vi "Signal State Controller.vi"(6 "stop":bool, 7 "reset":bool, 8 "error IO":errorcluster, 10 "current time":timestamp, 11 "signal configuration":refnum<class "SV Signal.lvclass">) -> (0 "error out":errorcluster, 1 "waveform dt":dbl, 2 "waveform t0":timestamp, 3 "signal configuration":refnum<class "SV Signal.lvclass">)   [LabVIEW 2017, in "SV Signal.lvclass"]
uses:
  <vilib>/addons/_NISVFA/_Generation/Signal Generation/SV Signal/SV Signal.lvclass
  <vilib>/addons/_NISVFA/_Generation/Signal Generation/SV Signal/SV Signal.lvclass/SV Signal.ctl
  <vilib>/addons/_NISVFA/_Generation/Signal Generation/SV Signal/sv_Signal State Attribute.ctl
  <vilib>/addons/_NISVFA/_Generation/Signal Generation/SV Signal/sv_Generation State.ctl
  <vilib>/addons/_NISVFA/_Generation/subVIs/sv_Optimum Location.ctl
  <vilib>/addons/_NISVFA/_Generation/SoundVib_Generation.lvlib
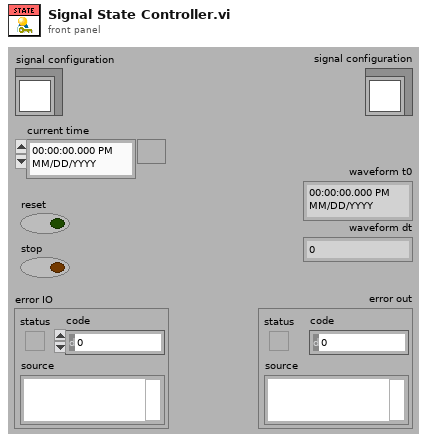
[diagram p1: front panel]
types:
  T1 = typedef "SV Signal.lvclass/sv_Signal State Attribute.ctl" = string
  T2 = typedef "SV Signal.lvclass/sv_Generation State.ctl" = enum16{"Idle", "Ramp Up", "Pre-Measurement Settling", "Measurement", "Post-Measurement Settling", "Discrete Sweep Transition", "Ramp Down", "Update"}
  T3 = typedef "SoundVib_Generation.lvlib/sv_Optimum Location.ctl" = enum16{"Zero Crossing, First Available", "Zero Crossing, Positive Slope", "Zero Crossing, Negative Slope", "Peak or Valley", "Peak", "Valley"}
  T4 = typedef "SV Signal.lvclass/sv_System Timing Model.ctl" = i64
  T5 = cluster{"system timing model":T4, "state":cluster{"RESET":bool, "generator timestamp":timestamp, "elapsed seconds":dbl, "elapsed samples":u64, "generation state":T2, "time offset at state":dbl, "samples generated at state":u64, "signal state":variant}, "duration of state":dbl, "samples remaining at state":i32}
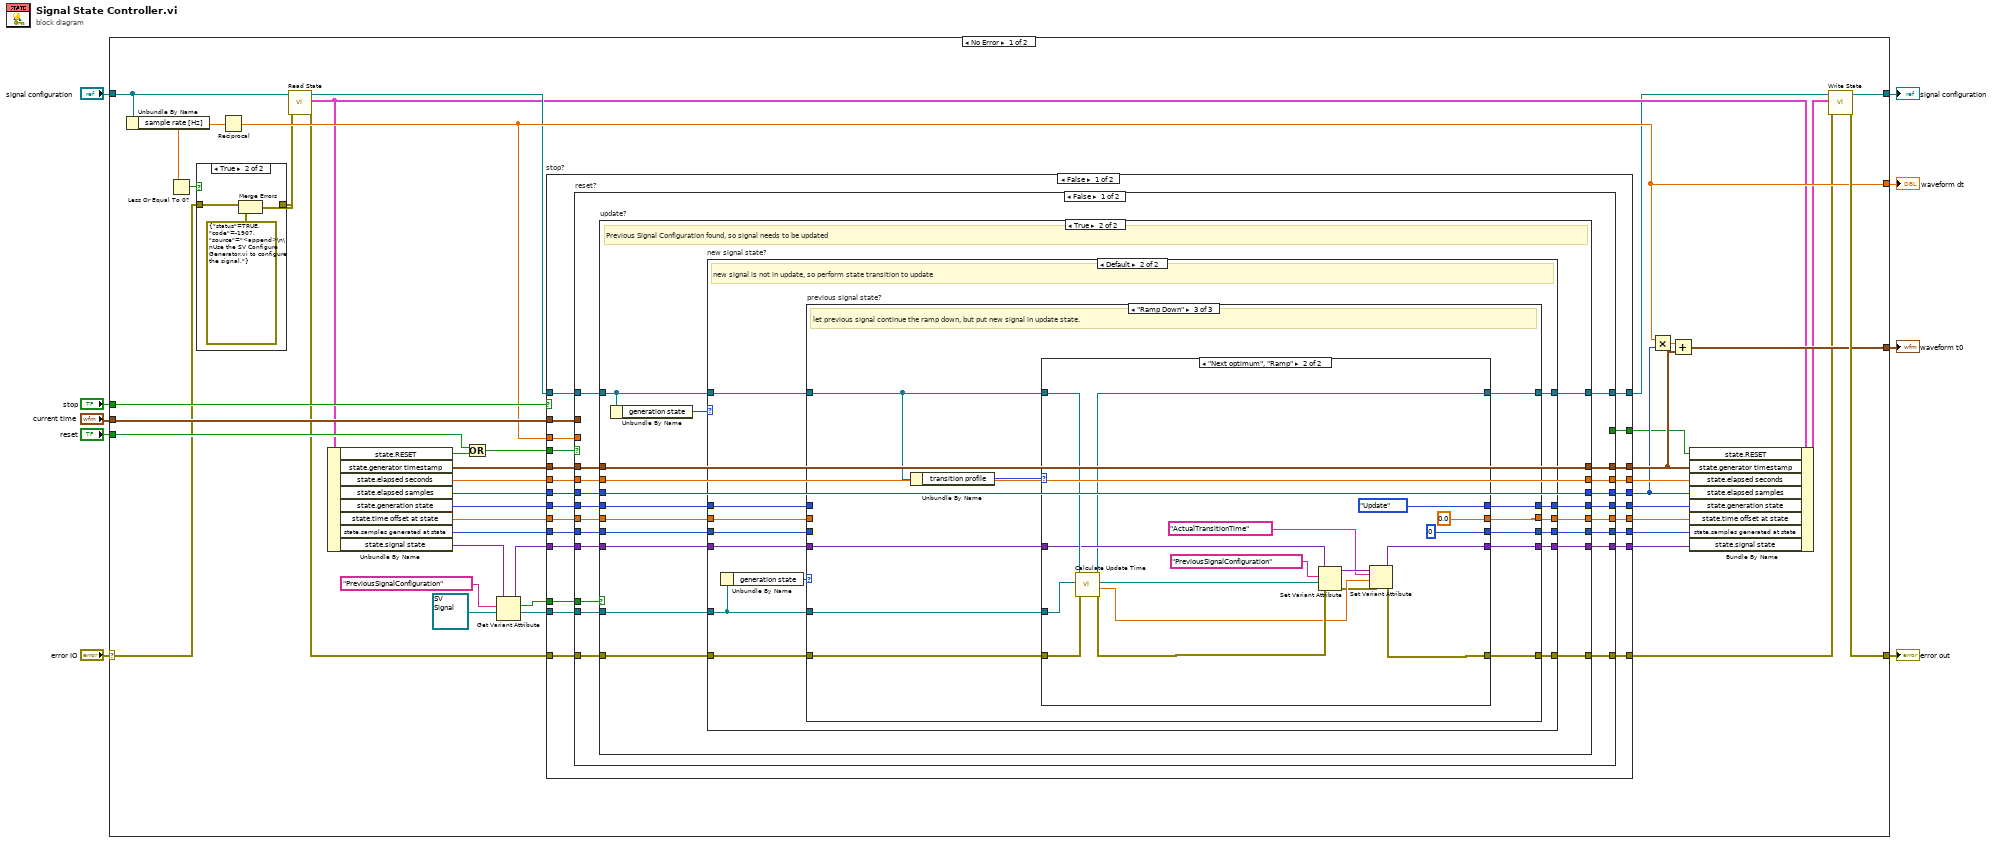
[diagram p0: block diagram]
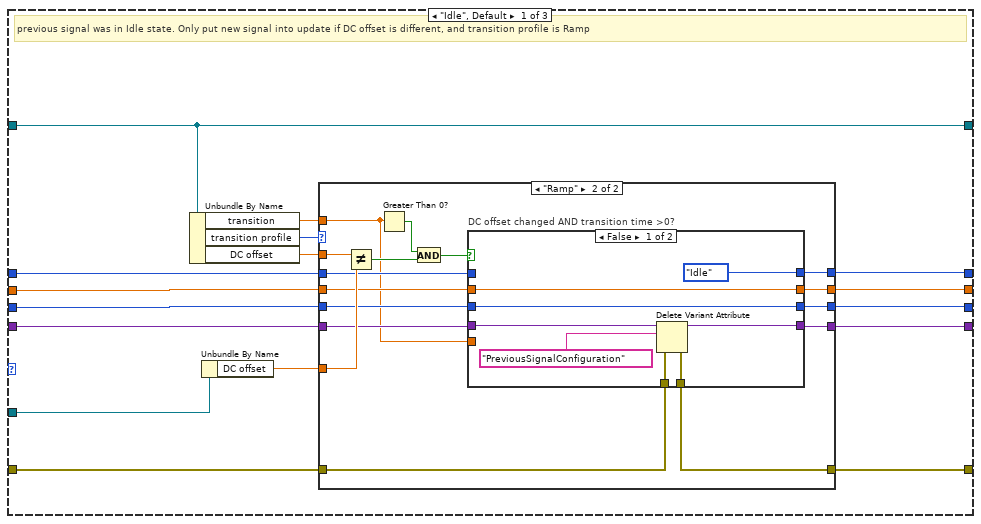
[diagram p5: hidden frame]
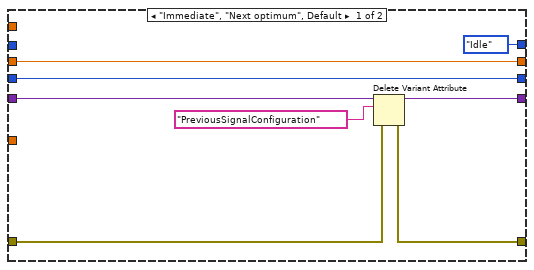
[diagram p6: hidden frame]
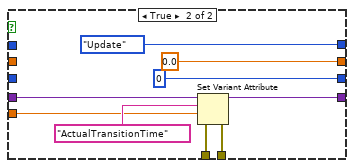
[diagram p7: hidden frame]
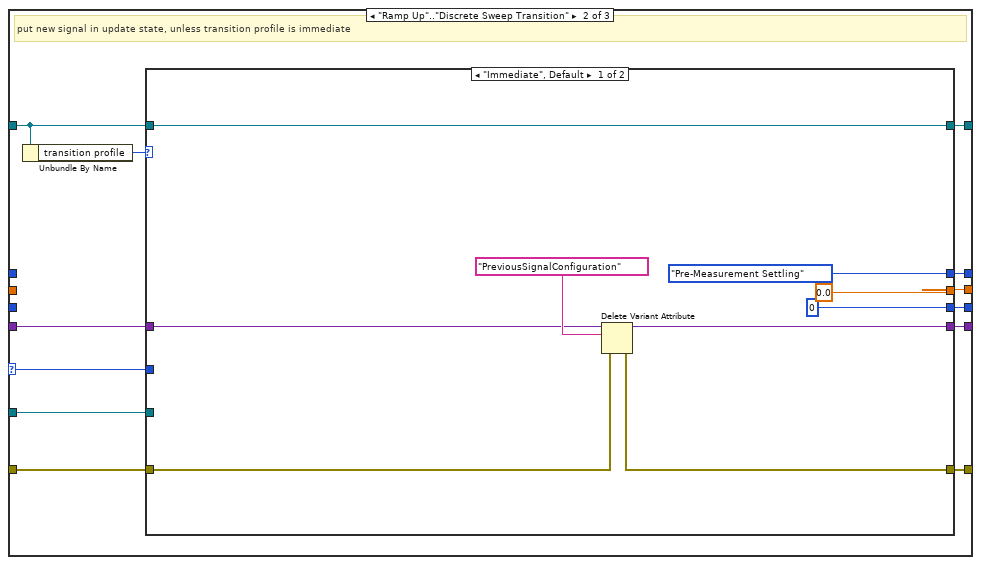
[diagram p8: hidden frame]
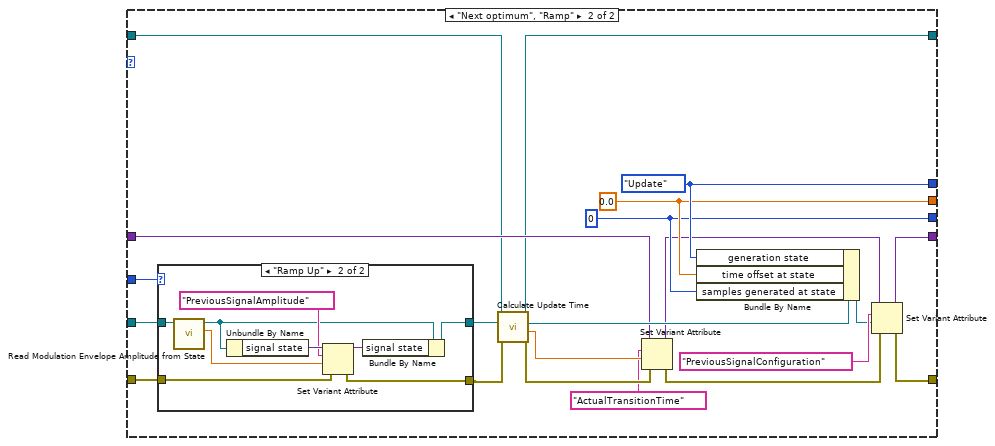
[diagram p9: hidden frame]
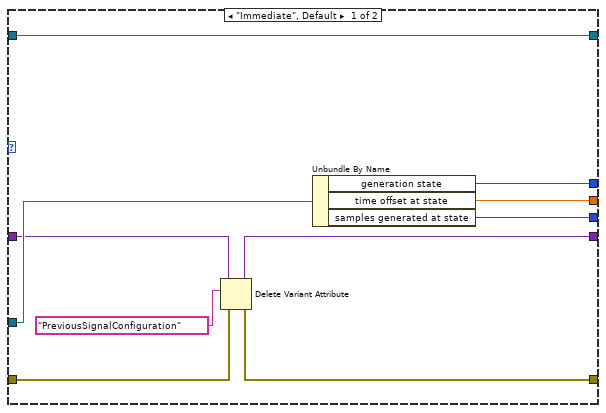
[diagram p11: hidden frame]
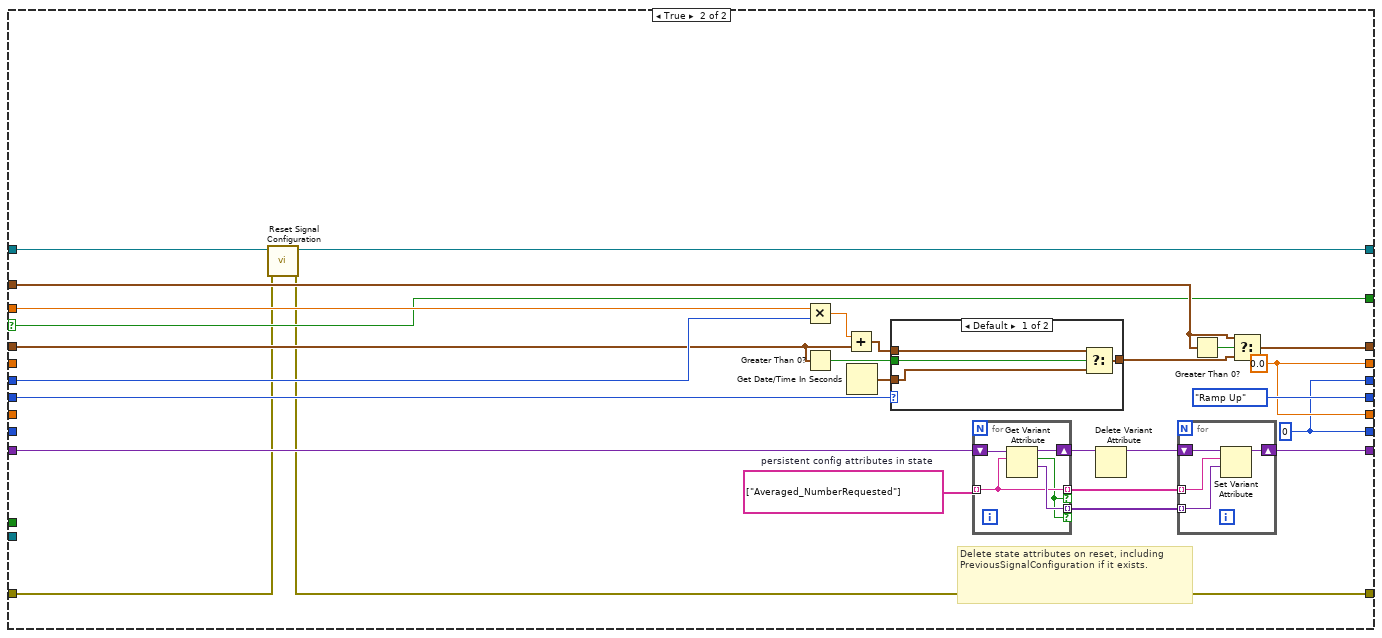
[diagram p12: hidden frame]
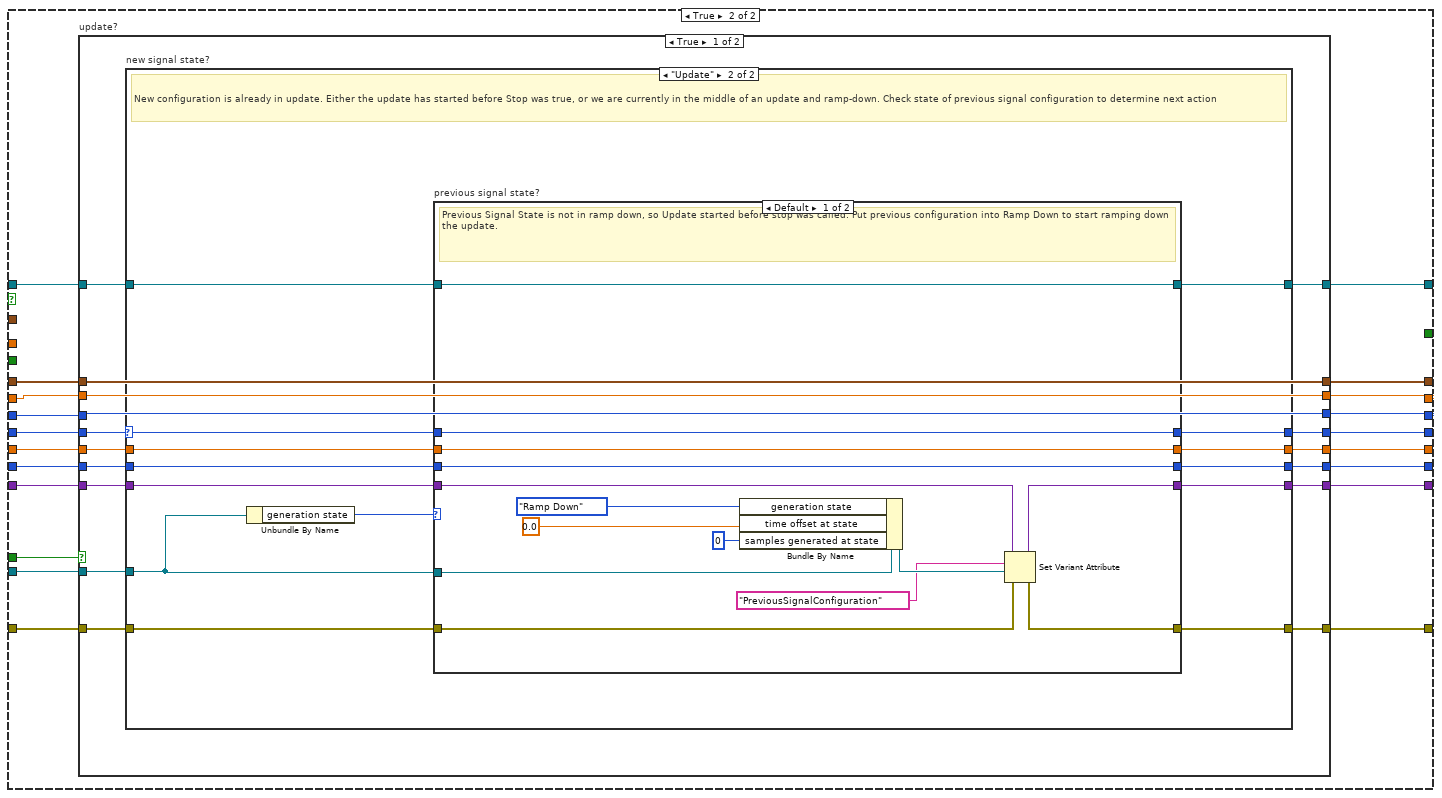
[diagram p14: hidden frame]
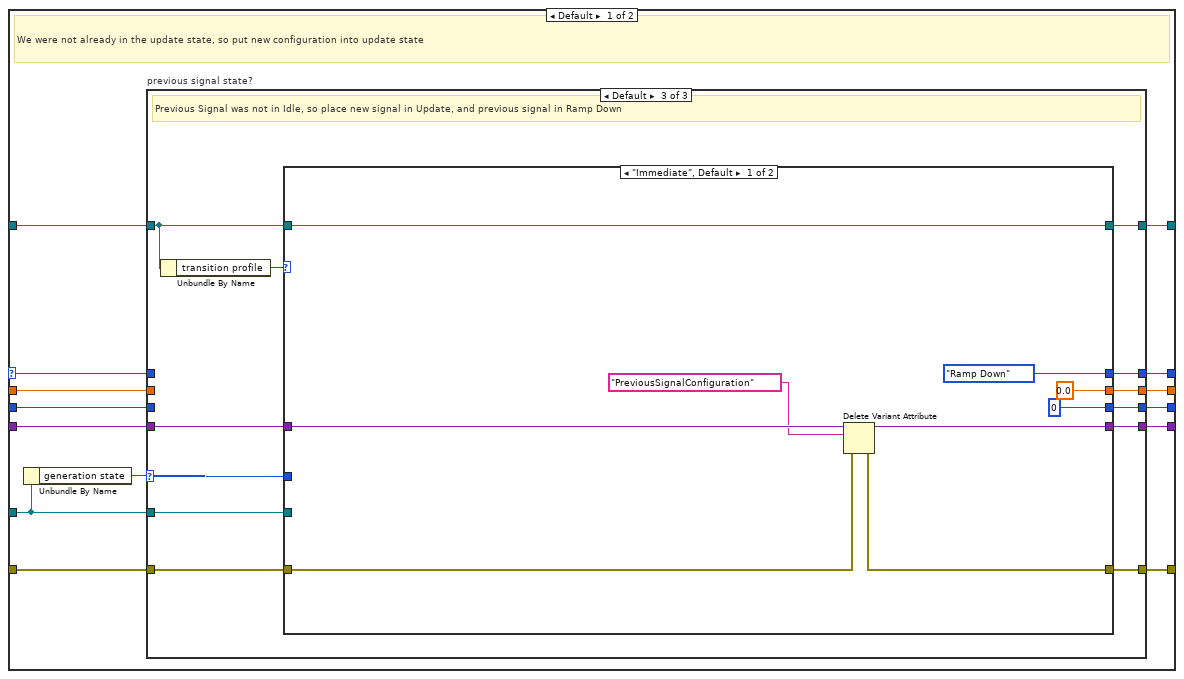
[diagram p15: hidden frame]
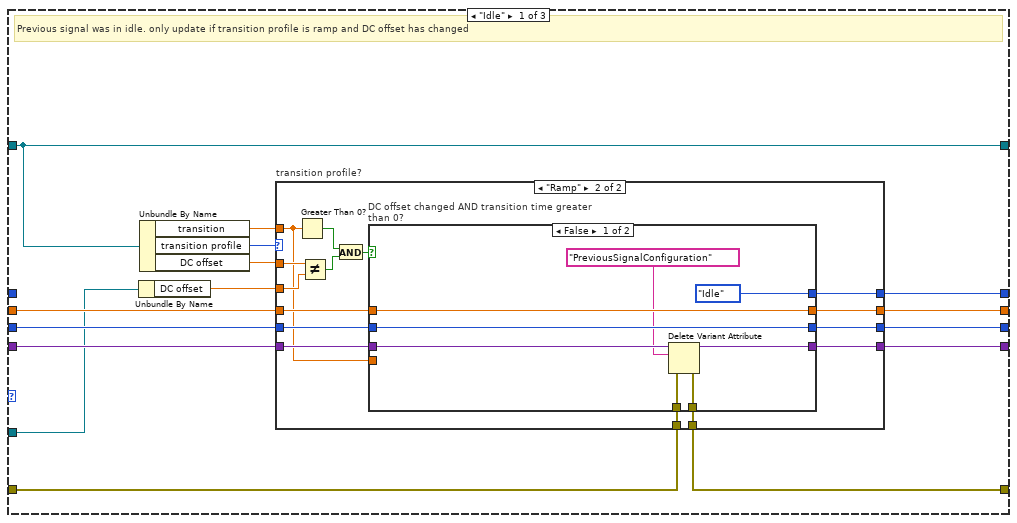
[diagram p16: hidden frame]
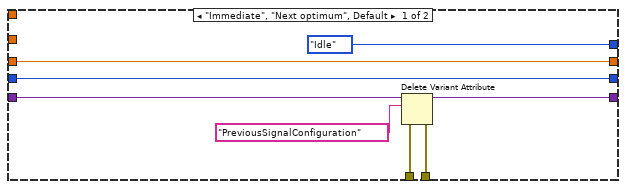
[diagram p17: hidden frame]
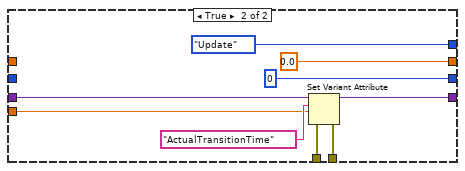
[diagram p18: hidden frame]
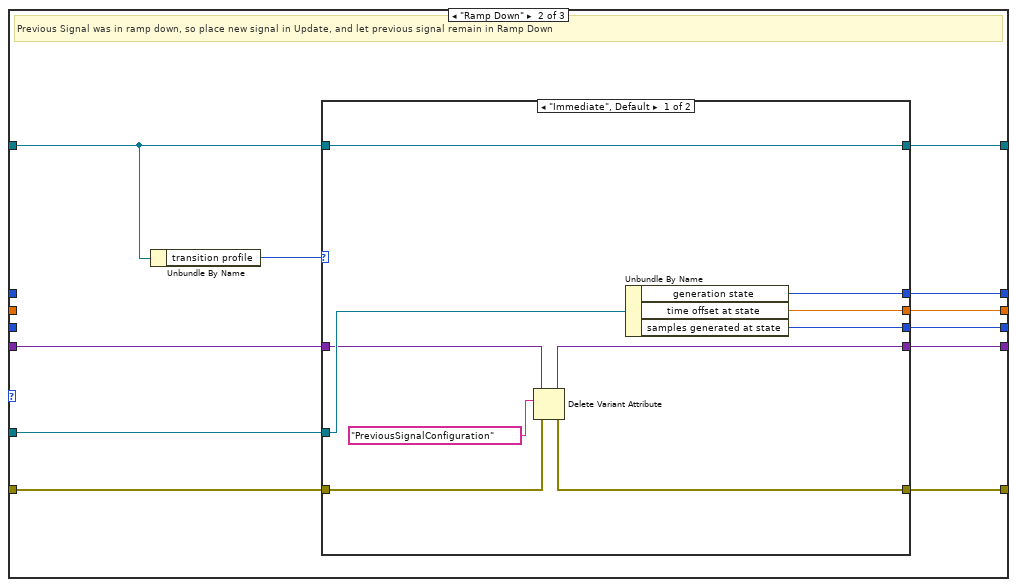
[diagram p19: hidden frame]
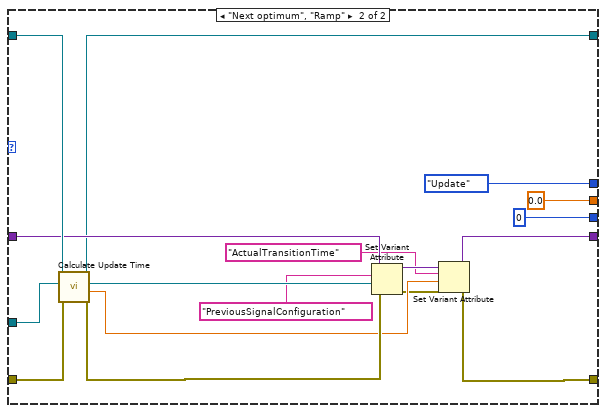
[diagram p20: hidden frame]
diagram:
  n1 = case shown="No Error" "error IO" {
    selector: "error IO" -> [w11 w618]
    tunnel: [w30 _] -> w9
    tunnel: "signal configuration" -> [w13 w619]
    tunnel: [w18 w619] -> w7
    tunnel: [w39 w618] -> w6
    tunnel: "stop" -> [w38 _]
    tunnel: "reset" -> [w36 _]
    tunnel: "current time" -> [w31 _]
    tunnel: [w29 nan] -> w1
    frame No Error {
      n2 = Unbundle By Name(w13) -> ("sample rate [Hz]"=w15:dbl)
      n3 = Less Or Equal To 0?(x=w15) -> (x <= 0?=w14:bool)
      n4 = case shown="True" w14 {
        tunnel: w11 -> [w51 w54]
        tunnel: [w51 w52] -> w10
        frame False {
        }
        frame True {
          n5 = Merge Errors(w54, errorcluster {"status"=TRUE, "code"=-1907, "source"="<append>\n\nUse the SV Configure Generator.vi to configure the signal."} ("error in (no error)")) -> (w52:errorcluster)
        }
      }
      n6 = Reciprocal(x=w15) -> (1/x=w29:dbl)
      n7 = call <vilib>:"Read State.vi"("error in (no error)"=w10, "signal configuration"=w13) -> ("error out"=w12:errorcluster, "generator state"=w20:T5, "signal configuration"=w28:refnum<class "SV Signal.lvclass">)  [unwired: 7 in]
      n8 = Unbundle By Name(w20) -> ("state.RESET"=w37:bool, "state.generator timestamp"=w44:timestamp, "state.elapsed seconds"=w45:dbl, "state.elapsed samples"=w46:u64, "state.generation state"=w47:T2, "state.time offset at state"=w43:dbl, "state.samples generated at state"=w42:u64, "state.signal state"=w25:variant)
      n9 = Or(x=w36, y=w37) -> (x .or. y?=w35:bool)
      n10 = Get Variant Attribute(Variant=w25, name=T1 "PreviousSignalConfiguration", default value (empty Variant)=refnum<class "SV Signal.lvclass"> refnum ("signal configuration")) -> (duplicate Variant=w24:variant, found=w23:bool, value=w22:refnum<class "SV Signal.lvclass">)  [unwired: 1 in, 1 out]
      n11 = case "stop?" shown="False" w38 {
        tunnel: [w78 w340] -> w50
        tunnel: [w77 w342] -> w49
        tunnel: [w76 w353] -> w48
        tunnel: [w75 w338] -> w32
        tunnel: w35 -> [w74 _]
        tunnel: w47 -> [w73 w350]
        tunnel: w46 -> [w72 w337]
        tunnel: w45 -> [w71 w339]
        tunnel: w44 -> [w70 w341]
        tunnel: w43 -> [w69 w349]
        tunnel: w42 -> [w68 w348]
        tunnel: [w67 w352] -> w41
        tunnel: [w66 w351] -> w40
        tunnel: w24 -> [w65 w347]
        tunnel: [w64 w346] -> w34
        tunnel: w31 -> [w63 _]
        tunnel: w29 -> [w62 _]
        tunnel: w28 -> [w57 w345]
        tunnel: w23 -> [w61 w336]
        tunnel: w22 -> [w60 w335]
        tunnel: w12 -> [w59 w343]
        tunnel: [w58 w344] -> w21
        tunnel: [w56 _] -> w17
        tunnel: [w55 w334] -> w16
        frame False {
          n12 = case "reset?" shown="False" w74 {
            selector: w74 -> [_ w297]
            tunnel: w70 -> [w95 w301]
            tunnel: [w96 w315] -> w77
            tunnel: [w94 w318] -> w78
            tunnel: [w92 w317] -> w75
            tunnel: w71 -> [w93 _]
            tunnel: w72 -> [w91 w304]
            tunnel: w73 -> [w89 w302]
            tunnel: [w90 sv_Generation_State."Ramp Up" ("generation state")] -> w76
            tunnel: w69 -> [w87 _]
            tunnel: w68 -> [w85 _]
            tunnel: [w88 w318] -> w67
            tunnel: [w86 w317] -> w66
            tunnel: w65 -> [w83 w309]
            tunnel: [w84 w308] -> w64
            tunnel: w63 -> [_ w314]
            tunnel: w62 -> [_ w305]
            tunnel: w61 -> [w97 _]
            tunnel: w60 -> [w98 _]
            tunnel: w59 -> [w82 w294]
            tunnel: [w81 w293] -> w58
            tunnel: w57 -> [w80 w296]
            tunnel: [_ w297] -> w56
            tunnel: [w79 w295] -> w55
            frame False {
              n13 = case "update?" shown="True" w97 {
                tunnel: w98 -> [_ w120]
                tunnel: [w107 w124] -> w96
                tunnel: w95 -> [w107 w124]
                tunnel: [w106 w123] -> w94
                tunnel: w93 -> [w106 w123]
                tunnel: [w105 w122] -> w92
                tunnel: w91 -> [w105 w122]
                tunnel: [w104 w114] -> w90
                tunnel: w89 -> [w104 w118]
                tunnel: [w103 w113] -> w88
                tunnel: w87 -> [w103 w117]
                tunnel: [w102 w112] -> w86
                tunnel: w85 -> [w102 w116]
                tunnel: [w101 w111] -> w84
                tunnel: w83 -> [w101 w115]
                tunnel: w82 -> [w100 w121]
                tunnel: [w100 w119] -> w81
                tunnel: w80 -> [w99 w110]
                tunnel: [w99 w108] -> w79
                frame False {
                  # "No previous signal configuration found, don't update signal state"
                }
                frame True {
                  # "Previous Signal Configuration found, so signal needs to be updated"
                  n14 = Unbundle By Name(w110) -> ("generation state"=w109:T2)
                  n15 = case "new signal state?" shown="Default" w109 {
                    tunnel: w121 -> [w130 w143]
                    tunnel: w120 -> [_ w142]
                    tunnel: [w130 w141] -> w119
                    tunnel: [w126 w140] -> w114
                    tunnel: w118 -> [w126 w139]
                    tunnel: [w127 w138] -> w113
                    tunnel: w117 -> [w127 w137]
                    tunnel: [w128 w136] -> w112
                    tunnel: w116 -> [w128 w135]
                    tunnel: [w129 w134] -> w111
                    tunnel: w115 -> [w129 w133]
                    tunnel: w110 -> [w125 w132]
                    tunnel: [w125 w131] -> w108
                    frame "Update" {
                      # "new signal already in update, so there is no need to change the state."
                    }
                    frame Default {
                      # "new signal is not in update, so perform state transition to update"
                      n16 = Unbundle By Name(w142) -> ("generation state"=w144:T2)
                      n17 = case "previous signal state?" shown="\"Ramp Down\"" w144 {
                        selector: w144 -> [_ w204 _]
                        tunnel: w143 -> [w148 w208 w261]
                        tunnel: w142 -> [w159 w209 w262]
                        tunnel: [w147 w207 w256] -> w141
                        tunnel: [w152 w206 w257] -> w140
                        tunnel: w139 -> [w156 _ _]
                        tunnel: [w151 w213 w258] -> w138
                        tunnel: w137 -> [w155 _ _]
                        tunnel: [w150 w212 w259] -> w136
                        tunnel: w135 -> [w154 _ _]
                        tunnel: [w149 w210 w260] -> w134
                        tunnel: w133 -> [w153 w211 w263]
                        tunnel: w132 -> [w145 w203 w264]
                        tunnel: [w145 w202 w255] -> w131
                        frame "Idle", Default {
                          # "previous signal was in Idle state. Only put new signal into update if DC offset is different, and transition profile is Ramp"
                          n18 = Unbundle By Name(w145) -> ("transition"=w146:dbl, "transition profile"=w160:enum16{"Immediate", "Next optimum", "Ramp"}, "DC offset"=w158:dbl)
                          n19 = Unbundle By Name(w159) -> ("DC offset"=w157:dbl)
                          n20 = case shown="\"Ramp\"" w160 {
                            tunnel: w158 -> [_ w184]
                            tunnel: w157 -> [_ w183]
                            tunnel: w156 -> [_ w182]
                            tunnel: w155 -> [w168 w181]
                            tunnel: w154 -> [w167 w180]
                            tunnel: w153 -> [w164 w179]
                            tunnel: [sv_Generation_State."Idle" ("generation state") w178] -> w152
                            tunnel: [w168 w177] -> w151
                            tunnel: [w167 w176] -> w150
                            tunnel: [w163 w175] -> w149
                            tunnel: w148 -> [w162 w174]
                            tunnel: [w161 w173] -> w147
                            tunnel: w146 -> [_ w169]
                            frame "Immediate", "Next optimum", Default {
                              n21 = Delete Variant Attribute(4:w162, 6:T1 "PreviousSignalConfiguration" ("name"), 7:w164) -> (0:w161:errorcluster, 3:w163:variant)  [unwired: 1 out]
                            }
                            frame "Ramp" {
                              n22 = Not Equal?(x=w184, y=w183) -> (x != y?=w171:bool)
                              n23 = Greater Than 0?(x=w169) -> (x > 0?=w172:bool)
                              n24 = And(x=w172, y=w171) -> (x .and. y?=w170:bool)
                              n25 = case "DC offset changed AND transition time >0?" shown="False" w170 {
                                tunnel: [sv_Generation_State."Idle" ("generation state") sv_Generation_State."Update" ("generation state")] -> w178
                                tunnel: [w191 0.0 ("time offset at state")] -> w177
                                tunnel: [w190 u64 0 ("samples generated at state")] -> w176
                                tunnel: w181 -> [w191 _]
                                tunnel: w180 -> [w190 _]
                                tunnel: [w188 w196] -> w175
                                tunnel: w179 -> [w189 w197]
                                tunnel: w174 -> [w186 w195]
                                tunnel: [w185 w194] -> w173
                                tunnel: w182 -> [_ _]
                                tunnel: w169 -> [_ w193]
                                frame False {
                                n26 = Delete Variant Attribute(4:w186, 6:T1 "PreviousSignalConfiguration" ("name"), 7:w189) -> (0:w185:errorcluster, 3:w188:variant)  [unwired: 1 out]
                                }
                                frame True {
                                n27 = Set Variant Attribute(Variant=w197, name=T1 "ActualTransitionTime" ("attribute"), value=w193, error in=w195) -> (Variant out=w196:variant, error out=w194:errorcluster)  [unwired: 1 out]
                                }
                              }
                            }
                          }
                        }
                        frame "Ramp Up".."Discrete Sweep Transition" {
                          # "put new signal in update state, unless transition profile is immediate"
                          n28 = Unbundle By Name(w203) -> ("transition profile"=w205:enum16{"Immediate", "Next optimum", "Ramp"})
                          n29 = case shown="\"Immediate\", Default" w205 {
                            tunnel: [0.0 ("TimeSinceLastReset") w236] -> w213
                            tunnel: [u64 0 ("elapsed samples") w235] -> w212
                            tunnel: w211 -> [w218 w232]
                            tunnel: [w217 w234] -> w210
                            tunnel: w209 -> [_ w242]
                            tunnel: w208 -> [w216 w241]
                            tunnel: [w215 w233] -> w207
                            tunnel: [sv_Generation_State."Pre-Measurement Settling" ("state.generation state") w237] -> w206
                            tunnel: w204 -> [_ w243]
                            tunnel: w203 -> [w214 w230]
                            tunnel: [w214 w223] -> w202
                            frame "Immediate", Default {
                              n30 = Delete Variant Attribute(4:w216, 6:T1 "PreviousSignalConfiguration" ("name"), 7:w218) -> (0:w215:errorcluster, 3:w217:variant)  [unwired: 1 out]
                            }
                            frame "Next optimum", "Ramp" {
                              w235 = u64 0 ("elapsed samples")
                              w236 = 0.0 ("TimeSinceLastReset")
                              w237 = sv_Generation_State."Update" ("generation state")
                              n31 = case shown="\"Ramp Up\"" w243 {
                                tunnel: w242 -> [w245 w254]
                                tunnel: [w245 w249] -> w231
                                tunnel: w241 -> [w244 w247]
                                tunnel: [w244 w246] -> w229
                                frame "Idle", Default {
                                }
                                frame "Ramp Up" {
                                n32 = call <vilib>:"Read Modulation Envelope Amplitude from State.vi"("SV Signal in"=w254) -> ("modulation envelope amplitude"=w251:dbl, "SV Signal out"=w250:refnum<class "SV Signal.lvclass">)  [unwired: 8 in, 1 out]
                                n33 = Unbundle By Name(w250) -> ("signal state"=w253:variant)
                                n34 = Set Variant Attribute(Variant=w253, name=T1 "PreviousSignalAmplitude" ("attribute"), value=w251, error in=w247) -> (Variant out=w248:variant, error out=w246:errorcluster)  [unwired: 1 out]
                                n35 = Bundle By Name(cluster=w250, "signal state"=w248) -> (w249:refnum<class "SV Signal.lvclass">)
                                }
                              }
                              n36 = call <vilib>:"Calculate Update Time.vi"("error in (no error)"=w229, "previous configuration in"=w231, "new configuration in"=w230) -> ("error out"=w238:errorcluster, "actual transition time"=w240:dbl, "previous configuration out"=w239:refnum<class "SV Signal.lvclass">, "new configuration out"=w223:refnum<class "SV Signal.lvclass">)  [unwired: 5 in]
                              n37 = Set Variant Attribute(Variant=w232, name=T1 "ActualTransitionTime" ("attribute"), value=w240, error in=w238) -> (Variant out=w226:variant, error out=w225:errorcluster)  [unwired: 1 out]
                              n38 = Bundle By Name(cluster=w239, "generation state"=w237, "time offset at state"=w236, "samples generated at state"=w235) -> (w227:refnum<class "SV Signal.lvclass">)
                              n39 = Set Variant Attribute(Variant=w226, name=T1 "PreviousSignalConfiguration" ("attribute"), value=w227, error in=w225) -> (Variant out=w234:variant, error out=w233:errorcluster)  [unwired: 1 out]
                            }
                          }
                        }
                        frame "Ramp Down" {
                          # "let previous signal continue the ramp down, but put new signal in update state."
                          n40 = Unbundle By Name(w264) -> ("transition profile"=w265:enum16{"Immediate", "Next optimum", "Ramp"})
                          n41 = case shown="\"Next optimum\", \"Ramp\"" w265 {
                            tunnel: [w274 sv_Generation_State."Update" ("generation state")] -> w257
                            tunnel: [w273 0.0 ("TimeSinceLastReset")] -> w258
                            tunnel: [w272 u64 0 ("elapsed samples")] -> w259
                            tunnel: [w267 w287] -> w260
                            tunnel: w263 -> [w268 w286]
                            tunnel: w262 -> [w275 w282]
                            tunnel: w264 -> [w266 w289]
                            tunnel: w261 -> [w270 w288]
                            tunnel: [w271 w284] -> w256
                            tunnel: [w266 w276] -> w255
                            frame "Immediate", Default {
                              n42 = Delete Variant Attribute(4:w270, 6:T1 "PreviousSignalConfiguration" ("attribute"), 7:w268) -> (0:w271:errorcluster, 3:w267:variant)  [unwired: 1 out]
                              n43 = Unbundle By Name(w275) -> ("generation state"=w274:T2, "time offset at state"=w273:dbl, "samples generated at state"=w272:u64)
                            }
                            frame "Next optimum", "Ramp" {
                              n44 = call <vilib>:"Calculate Update Time.vi"("error in (no error)"=w288, "previous configuration in"=w282, "new configuration in"=w289) -> ("error out"=w285:errorcluster, "actual transition time"=w281:dbl, "previous configuration out"=w283:refnum<class "SV Signal.lvclass">, "new configuration out"=w276:refnum<class "SV Signal.lvclass">)  [unwired: 5 in]
                              n45 = Set Variant Attribute(Variant=w286, name=T1 "PreviousSignalConfiguration" ("attribute"), value=w283, error in=w285) -> (Variant out=w278:variant, error out=w279:errorcluster)  [unwired: 1 out]
                              n46 = Set Variant Attribute(Variant=w278, name=T1 "ActualTransitionTime" ("attribute"), value=w281, error in=w279) -> (Variant out=w287:variant, error out=w284:errorcluster)  [unwired: 1 out]
                            }
                          }
                        }
                      }
                    }
                  }
                }
              }
            }
            frame True {
              w298 = T1[] ["Averaged_NumberRequested"]  # persistent config attributes in state
              w317 = u64 0 ("elapsed samples")
              w318 = 0.0 ("TimeSinceLastReset")
              # "Delete state attributes on reset, including PreviousSignalConfiguration if it exists."
              n47 = call-dynamic "Reset Signal Configuration.vi"("error in (no error)"=w294, "signal configuration in"=w296) -> ("error out"=w293:errorcluster, "signal configuration out"=w295:refnum<class "SV Signal.lvclass">)  [unwired: 8 in]
              n48 = Multiply(x=w305, y=w304) -> (x*y=w300:dbl)
              n49 = Greater Than 0?(x=w301) -> (x > 0?=w307:bool)
              n50 = Add(x=w300, y=w301) -> (x+y=w299:timestamp)
              n51 = Get Date/Time In Seconds() -> (seconds since 1Jan1904=w306:timestamp)
              n52 = case shown="Default" w302 {
                tunnel: w307 -> [w323 _]
                tunnel: w306 -> [w322 w324]
                tunnel: [w321 w324] -> w303
                tunnel: w299 -> [w320 _]
                frame Default {
                  n53 = Select(t=w320, s=w323, f=w322) -> (s? t:f=w321:timestamp)
                }
                frame "Idle" {
                }
              }
              n54 = for {
                tunnel: w298 -> [w330] mode=indexing
                shift-right: [w332] -> w313
                shift-left: w309 -> [w333]
                tunnel: [w331] -> w310 mode=indexing if=w329
                tunnel: [w330] -> w311 mode=indexing if=w329
                n55 = Get Variant Attribute(Variant=w333, name=w330) -> (duplicate Variant=w332:variant, found=w329:bool, value=w331:variant)  [unwired: 2 in, 1 out]
              }
              n56 = Delete Variant Attribute(7:w313) -> (3:w312:variant)  [unwired: 2 in, 2 out]
              n57 = for {
                tunnel: w310 -> [w326] mode=indexing
                shift-right: [w328] -> w308
                shift-left: w312 -> [w327]
                tunnel: w311 -> [w325] mode=indexing
                n58 = Set Variant Attribute(Variant=w327, name=w325, value=w326) -> (Variant out=w328:variant)  [unwired: 1 in, 2 out]
              }
              n59 = Greater Than 0?(x=w314) -> (x > 0?=w316:bool)
              n60 = Select(t=w314, s=w316, f=w303) -> (s? t:f=w315:timestamp)
            }
          }
        }
        frame True {
          n61 = case "update?" shown="True" w336 {
            tunnel: [w369 w578] -> w353
            tunnel: [w368 w577] -> w352
            tunnel: [w367 w576] -> w351
            tunnel: w350 -> [w356 w575]
            tunnel: w349 -> [w366 w574]
            tunnel: w348 -> [w365 w573]
            tunnel: w347 -> [w364 w572]
            tunnel: [w363 w571] -> w346
            tunnel: w345 -> [w355 w565]
            tunnel: [w362 w570] -> w344
            tunnel: w343 -> [w361 w569]
            tunnel: [w360 w568] -> w342
            tunnel: w341 -> [w360 w568]
            tunnel: [w359 w567] -> w340
            tunnel: w339 -> [w359 w567]
            tunnel: [w358 w566] -> w338
            tunnel: w337 -> [w358 w566]
            tunnel: w335 -> [w357 _]
            tunnel: [w354 w565] -> w334
            frame True {
              n62 = case "new signal state?" shown="\"Update\"" w356 {
                selector: w356 -> [w371 w537]
                tunnel: [w383 w538] -> w369
                tunnel: [w382 w535] -> w368
                tunnel: [w381 w534] -> w367
                tunnel: w366 -> [w380 w536]
                tunnel: w365 -> [w379 w533]
                tunnel: w364 -> [w378 w540]
                tunnel: [w377 w539] -> w363
                tunnel: w355 -> [w376 w532]
                tunnel: [w375 w543] -> w362
                tunnel: w361 -> [w374 w542]
                tunnel: w357 -> [w373 w541]
                tunnel: [w370 w531] -> w354
                frame Default {
                  # "We were not already in the update state, so put new configuration into update state"
                  n63 = Unbundle By Name(w373) -> ("generation state"=w372:T2)
                  n64 = case "previous signal state?" shown="Default" w372 {
                    selector: w372 -> [_ _ w479]
                    tunnel: [w397 w449 w488] -> w383
                    tunnel: [w396 w448 w481] -> w382
                    tunnel: [w394 w447 w482] -> w381
                    tunnel: w380 -> [w395 _ _]
                    tunnel: w379 -> [w393 _ _]
                    tunnel: w378 -> [w391 w445 w487]
                    tunnel: [w392 w446 w486] -> w377
                    tunnel: w376 -> [w384 w442 w478]
                    tunnel: [w386 w440 w485] -> w375
                    tunnel: w374 -> [w387 w441 w484]
                    tunnel: w373 -> [w390 w443 w483]
                    tunnel: w371 -> [_ _ _]
                    tunnel: [w384 w439 w477] -> w370
                    frame "Idle" {
                      # "Previous signal was in idle. only update if transition profile is ramp and DC offset has changed"
                      n65 = Unbundle By Name(w390) -> ("DC offset"=w388:dbl)
                      n66 = Unbundle By Name(w384) -> ("transition"=w385:dbl, "transition profile"=w398:enum16{"Immediate", "Next optimum", "Ramp"}, "DC offset"=w389:dbl)
                      n67 = case "transition profile?" shown="\"Ramp\"" w398 {
                        tunnel: [sv_Generation_State."Idle" ("generation state") w421] -> w397
                        tunnel: [w405 w420] -> w396
                        tunnel: w395 -> [w405 w416]
                        tunnel: [w404 w419] -> w394
                        tunnel: w393 -> [w404 w415]
                        tunnel: [w402 w414] -> w392
                        tunnel: w391 -> [w403 w413]
                        tunnel: w389 -> [_ w418]
                        tunnel: w388 -> [_ w417]
                        tunnel: w387 -> [w400 w412]
                        tunnel: [w399 w411] -> w386
                        tunnel: w385 -> [_ w407]
                        frame "Immediate", "Next optimum", Default {
                          n68 = Delete Variant Attribute(4:w400, 6:T1 "PreviousSignalConfiguration" ("name"), 7:w403) -> (0:w399:errorcluster, 3:w402:variant)  [unwired: 1 out]
                        }
                        frame "Ramp" {
                          n69 = Greater Than 0?(x=w407) -> (x > 0?=w410:bool)
                          n70 = Not Equal?(x=w418, y=w417) -> (x != y?=w409:bool)
                          n71 = And(x=w410, y=w409) -> (x .and. y?=w408:bool)
                          n72 = case "DC offset changed AND transition time greater than 0?" shown="False" w408 {
                            tunnel: [sv_Generation_State."Idle" ("generation state") sv_Generation_State."Update" ("generation state")] -> w421
                            tunnel: [w428 0.0 ("time offset at state")] -> w420
                            tunnel: [w427 u64 0 ("samples generated at state")] -> w419
                            tunnel: w416 -> [w428 _]
                            tunnel: w415 -> [w427 _]
                            tunnel: [w425 w433] -> w414
                            tunnel: w413 -> [w426 w434]
                            tunnel: w412 -> [w423 w432]
                            tunnel: [w422 w431] -> w411
                            tunnel: w407 -> [_ w430]
                            frame False {
                              n73 = Delete Variant Attribute(4:w423, 6:T1 "PreviousSignalConfiguration" ("name"), 7:w426) -> (0:w422:errorcluster, 3:w425:variant)  [unwired: 1 out]
                            }
                            frame True {
                              n74 = Set Variant Attribute(Variant=w434, name=T1 "ActualTransitionTime" ("attribute"), value=w430, error in=w432) -> (Variant out=w433:variant, error out=w431:errorcluster)  [unwired: 1 out]
                            }
                          }
                        }
                      }
                    }
                    frame "Ramp Down" {
                      # "Previous Signal was in ramp down, so place new signal in Update, and let previous signal remain in Ramp Down"
                      n75 = Unbundle By Name(w442) -> ("transition profile"=w444:enum16{"Immediate", "Next optimum", "Ramp"})
                      n76 = case shown="\"Immediate\", Default" w444 {
                        tunnel: [w458 sv_Generation_State."Update" ("generation state")] -> w449
                        tunnel: [w457 0.0 ("TimeSinceLastReset")] -> w448
                        tunnel: [w456 u64 0 ("elapsed samples")] -> w447
                        tunnel: [w451 w471] -> w446
                        tunnel: w445 -> [w452 w470]
                        tunnel: w443 -> [w459 w466]
                        tunnel: w442 -> [w450 w473]
                        tunnel: w441 -> [w454 w472]
                        tunnel: [w455 w468] -> w440
                        tunnel: [w450 w460] -> w439
                        frame "Immediate", Default {
                          n77 = Delete Variant Attribute(4:w454, 6:T1 "PreviousSignalConfiguration" ("attribute"), 7:w452) -> (0:w455:errorcluster, 3:w451:variant)  [unwired: 1 out]
                          n78 = Unbundle By Name(w459) -> ("generation state"=w458:T2, "time offset at state"=w457:dbl, "samples generated at state"=w456:u64)
                        }
                        frame "Next optimum", "Ramp" {
                          n79 = call <vilib>:"Calculate Update Time.vi"("error in (no error)"=w472, "previous configuration in"=w466, "new configuration in"=w473) -> ("error out"=w469:errorcluster, "actual transition time"=w465:dbl, "previous configuration out"=w467:refnum<class "SV Signal.lvclass">, "new configuration out"=w460:refnum<class "SV Signal.lvclass">)  [unwired: 5 in]
                          n80 = Set Variant Attribute(Variant=w470, name=T1 "PreviousSignalConfiguration" ("attribute"), value=w467, error in=w469) -> (Variant out=w462:variant, error out=w463:errorcluster)  [unwired: 1 out]
                          n81 = Set Variant Attribute(Variant=w462, name=T1 "ActualTransitionTime" ("attribute"), value=w465, error in=w463) -> (Variant out=w471:variant, error out=w468:errorcluster)  [unwired: 1 out]
                        }
                      }
                    }
                    frame Default {
                      # "Previous Signal was not in Idle, so place new signal in Update, and previous signal in Ramp Down"
                      n82 = Unbundle By Name(w478) -> ("transition profile"=w480:enum16{"Immediate", "Next optimum", "Ramp"})
                      n83 = case shown="\"Immediate\", Default" w480 {
                        tunnel: [sv_Generation_State."Ramp Down" ("generation state") sv_Generation_State."Update" ("generation state")] -> w488
                        tunnel: w487 -> [w494 w518]
                        tunnel: [w490 w517] -> w486
                        tunnel: [w491 w516] -> w485
                        tunnel: w484 -> [w492 w511]
                        tunnel: w483 -> [_ w512]
                        tunnel: [u64 0 ("elapsed samples") w515] -> w482
                        tunnel: [0.0 ("TimeSinceLastReset") w514] -> w481
                        tunnel: w479 -> [_ w513]
                        tunnel: w478 -> [w489 w506]
                        tunnel: [w489 w498] -> w477
                        frame "Immediate", Default {
                          n84 = Delete Variant Attribute(4:w492, 6:T1 "PreviousSignalConfiguration" ("name"), 7:w494) -> (0:w491:errorcluster, 3:w490:variant)  [unwired: 1 out]
                        }
                        frame "Next optimum", "Ramp" {
                          w515 = u64 0 ("elapsed samples")
                          w514 = 0.0 ("TimeSinceLastReset")
                          n85 = case shown="\"Ramp Up\"" w513 {
                            tunnel: w512 -> [w521 w530]
                            tunnel: [w521 w525] -> w508
                            tunnel: w511 -> [w520 w523]
                            tunnel: [w520 w522] -> w510
                            frame "Idle", Default {
                            }
                            frame "Ramp Up" {
                              n86 = call <vilib>:"Read Modulation Envelope Amplitude from State.vi"("SV Signal in"=w530) -> ("modulation envelope amplitude"=w527:dbl, "SV Signal out"=w526:refnum<class "SV Signal.lvclass">)  [unwired: 8 in, 1 out]
                              n87 = Unbundle By Name(w526) -> ("signal state"=w529:variant)
                              n88 = Set Variant Attribute(Variant=w529, name=T1 "PreviousSignalAmplitude" ("attribute"), value=w527, error in=w523) -> (Variant out=w524:variant, error out=w522:errorcluster)  [unwired: 1 out]
                              n89 = Bundle By Name(cluster=w526, "signal state"=w524) -> (w525:refnum<class "SV Signal.lvclass">)
                            }
                          }
                          n90 = call <vilib>:"Calculate Update Time.vi"("error in (no error)"=w510, "previous configuration in"=w508, "new configuration in"=w506) -> ("error out"=w509:errorcluster, "actual transition time"=w505:dbl, "previous configuration out"=w507:refnum<class "SV Signal.lvclass">, "new configuration out"=w498:refnum<class "SV Signal.lvclass">)  [unwired: 5 in]
                          n91 = Set Variant Attribute(Variant=w518, name=T1 "ActualTransitionTime" ("attribute"), value=w505, error in=w509) -> (Variant out=w501:variant, error out=w500:errorcluster)  [unwired: 1 out]
                          n92 = Bundle By Name(cluster=w507, "generation state"=sv_Generation_State."Ramp Down" ("state.generation state"), "time offset at state"=w514, "samples generated at state"=w515) -> (w502:refnum<class "SV Signal.lvclass">)
                          n93 = Set Variant Attribute(Variant=w501, name=T1 "PreviousSignalConfiguration" ("attribute"), value=w502, error in=w500) -> (Variant out=w517:variant, error out=w516:errorcluster)  [unwired: 1 out]
                        }
                      }
                    }
                  }
                }
                frame "Update" {
                  # "New configuration is already in update. Either the update has started before Stop was true, or we are currently in the middle of an update and ramp-down. Check state of previous signal configuration to determine next action"
                  n94 = Unbundle By Name(w541) -> ("generation state"=w544:T2)
                  n95 = case "previous signal state?" shown="Default" w544 {
                    tunnel: [w553 w564] -> w543
                    tunnel: w542 -> [w552 w564]
                    tunnel: w541 -> [w558 _]
                    tunnel: w540 -> [w551 w563]
                    tunnel: [w550 w563] -> w539
                    tunnel: [w548 w562] -> w538
                    tunnel: w537 -> [w548 w562]
                    tunnel: w536 -> [w547 w561]
                    tunnel: [w547 w561] -> w535
                    tunnel: [w546 w560] -> w534
                    tunnel: w533 -> [w546 w560]
                    tunnel: w532 -> [w545 w559]
                    tunnel: [w545 w559] -> w531
                    frame Default {
                      # "Previous Signal State is not in ramp down, so Update started before stop was called. Put previous configuration into Ramp Down to start ramping down the update."
                      n96 = Bundle By Name(cluster=w558, "generation state"=sv_Generation_State."Ramp Down" ("state.generation state"), "time offset at state"=0.0 ("state.time offset at state"), "samples generated at state"=u64 0 ("state.samples generated at state")) -> (w557:refnum<class "SV Signal.lvclass">)
                      n97 = Set Variant Attribute(Variant=w551, name=T1 "PreviousSignalConfiguration" ("attribute"), value=w557, error in=w552) -> (Variant out=w550:variant, error out=w553:errorcluster)  [unwired: 1 out]
                    }
                    frame "Ramp Down" {
                      # "Previous Signal State is already in ramp down, which means we are ramping down an updating signal. Continue updating and ramping down."
                    }
                  }
                }
              }
            }
            frame False {
              n98 = case shown="Default" w575 {
                selector: w575 -> [w583 w589]
                tunnel: [w583 sv_Generation_State."Ramp Down" ("generation state")] -> w578
                tunnel: [w582 0.0 ("TimeSinceLastReset")] -> w577
                tunnel: [w581 u64 0 ("elapsed samples")] -> w576
                tunnel: w574 -> [w582 _]
                tunnel: w573 -> [w581 _]
                tunnel: w572 -> [w580 w587]
                tunnel: [w580 w592] -> w571
                tunnel: w565 -> [_ w584]
                tunnel: [w579 w591] -> w570
                tunnel: w569 -> [w579 w586]
                frame "Idle", "Ramp Down" {
                }
                frame Default {
                  n99 = case shown="\"Ramp Up\"" w589 {
                    tunnel: [w597 w603] -> w588
                    tunnel: w587 -> [w597 w604]
                    tunnel: w586 -> [w596 w599]
                    tunnel: [w596 w602] -> w585
                    tunnel: w584 -> [_ w601]
                    frame "Idle", Default {
                    }
                    frame "Ramp Up" {
                      n100 = call <vilib>:"Read Modulation Envelope Amplitude from State.vi"("error in (no error)"=w599, "SV Signal in"=w601) -> ("error out"=w598:errorcluster, "modulation envelope amplitude"=w600:dbl)  [unwired: 7 in, 1 out]
                      n101 = Set Variant Attribute(Variant=w604, name=T1 "PreviousSignalAmplitude" ("attribute"), value=w600, error in=w598) -> (Variant out=w603:variant, error out=w602:errorcluster)  [unwired: 1 out]
                    }
                  }
                  n102 = Unbundle By Name(w584) -> ("transition profile"=w590:enum16{"Immediate", "Next optimum", "Ramp"})
                  n103 = case shown="\"Next optimum\"" w590 {
                    tunnel: w588 -> [w607 w616]
                    tunnel: [w607 w615] -> w592
                    tunnel: w585 -> [w606 w610]
                    tunnel: [w606 w609] -> w591
                    tunnel: w584 -> [_ w608]
                    frame "Immediate", Default {
                    }
                    frame "Next optimum" {
                      n104 = call-dynamic "Compute Optimal Transition Time.vi"("error in (no error)"=w610, "optimum"=sv_Optimum_Location."Zero Crossing, First Available", "SV Signal in"=w608) -> ("error out"=w611:errorcluster, "optimal transition time"=w612:dbl)  [unwired: 6 in, 1 out]
                      n105 = Set Variant Attribute(Variant=w616, name=T1 "OptimalTransitionTime" ("attribute"), value=w612, error in=w611) -> (Variant out=w615:variant, error out=w609:errorcluster)  [unwired: 1 out]
                    }
                  }
                }
              }
            }
          }
        }
      }
      n106 = Multiply(x=w29, y=w32) -> (x*y=w33:dbl)
      n107 = Add(x=w33, y=w49) -> (x+y=w30:timestamp)
      n108 = Bundle By Name(cluster=w20, "state.RESET"=w17, "state.generator timestamp"=w49, "state.elapsed seconds"=w50, "state.elapsed samples"=w32, "state.generation state"=w48, "state.time offset at state"=w41, "state.samples generated at state"=w40, "state.signal state"=w34) -> (w19:T5)
      n109 = call <vilib>:"Write State.vi"("error in (no error)"=w21, "generator state"=w19, "signal configuration"=w16) -> ("error out"=w39:errorcluster, "signal configuration"=w18:refnum<class "SV Signal.lvclass">)  [unwired: 7 in]
    }
    frame Error {
    }
  }
  "signal configuration" <- w7
  "error out" <- w6
  "waveform t0" <- w9
  "waveform dt" <- w1
